vi "uA_DAQ_Init_Monitor_Stream_vbat_selector.vi"(8 "error in (no error)":errorcluster, 9 "USB":tag, 10 "Ext PW Vol Monitor":bool, 11 "Refnum in":refnum<k21>) -> (0 "error out":errorcluster, 3 "Refnum out":refnum<k21>)   [LabVIEW 2015]
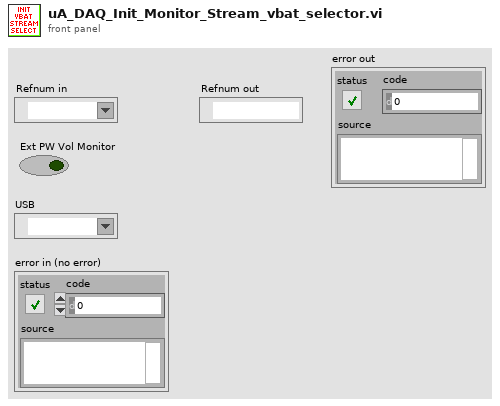
[diagram p1: front panel]
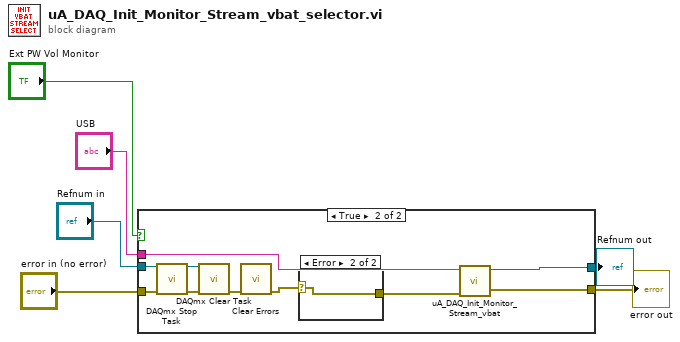
[diagram p0: block diagram]
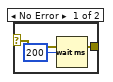
[diagram p3: hidden frame]
diagram:
  n1 = case shown="True" "Ext PW Vol Monitor" {
    tunnel: "USB" -> [_ w18]
    tunnel: "error in (no error)" -> [w7 w14]
    tunnel: "Refnum in" -> [w8 w13]
    tunnel: [w8 w17] -> w6
    tunnel: [w7 w11] -> w1
    frame False {
    }
    frame True {
      n2 = call <vilib>:"DAQmx Stop Task.vi"("task/channels in"=w13, "error in"=w14) -> ("task out"=w12:refnum<k21>, "error out"=w15:errorcluster)  [unwired: 12 in]
      n3 = call <vilib>:"DAQmx Clear Task.vi"("task in"=w12, "error in"=w15) -> ("error out"=w16:errorcluster)  [unwired: 13 in]
      n4 = call <vilib>:"Clear Errors.vi"("error in (no error)"=w16) -> ("error out"=w10:errorcluster)  [unwired: 5 in, 1 out]
      n5 = case shown="Error" w10 {
        selector: w10 -> [w20 w21]
        tunnel: [w20 w21] -> w9
        frame No Error {
          n6 = Wait (ms)(milliseconds to wait=u32 200) -> ()  [unwired: 1 out]
        }
        frame Error {
        }
      }
      n7 = call "uA_DAQ_Init_Monitor_Stream_vbat.vi"("error in (no error)"=w9, "USB"=w18) -> ("error out"=w11:errorcluster, "Refnum out"=w17:refnum<k21>)  [unwired: 8 in]
    }
  }
  "Refnum out" <- w6
  "error out" <- w1
